vi "PathPlanner_PathFinding_GetCurrentPath.vi"() -> (3 "NewPthAvailable":bool)   [LabVIEW 2019]
uses:
  PathPlanner_PathFinding_Globals.vi
  PathPlanner24.lvlib
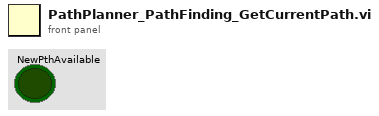
[diagram p1: front panel]
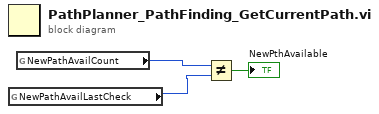
[diagram p0: block diagram]
diagram:
  n1 = global read "PathPlanner_PathFinding_Globals.vi" "NewPathAvailLastCheck"() -> (w2:i32)
  n2 = global read "PathPlanner_PathFinding_Globals.vi" "NewPathAvailCount"() -> (w3:i32)
  n3 = Not Equal?(x=w3, y=w2) -> (x != y?=→"NewPthAvailable":bool)
